vi "Read Unified Msg Set.vi"(11 "Attributes in":refnum<class "Attributes.lvclass">) -> (2 "Unified Msg Set":T1)   [LabVIEW 2020, in "jettl.lvlib" / "Attributes.lvlib" / "Attributes.lvclass"]
uses:
  Attributes.lvclass
  Msg/Msg.lvclass
  Actor/Msgs.ctl
  Actor/Actor.lvlib
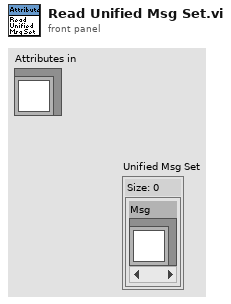
[diagram p1: front panel]
types:
  T1 = typedef "jettl.lvlib/Actor.lvlib/Msgs.ctl" = set{refnum<class "Msg.lvclass">}
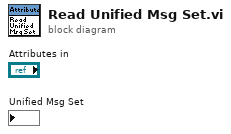
[diagram p0: block diagram]
diagram:
